vi "example-SetGetControlValue.vi"() -> ()   [LabVIEW 2020]
uses:
  SetGetControlValue.lvlib
panel:
  out "x = y? 2":bool
  out "x = y?":bool
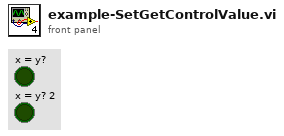
[diagram p1: front panel]
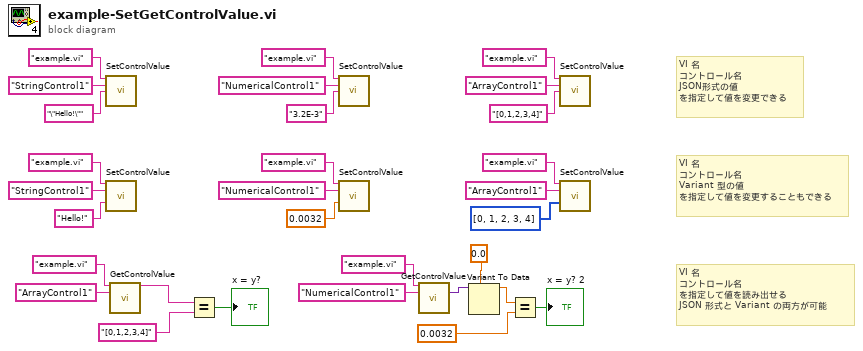
[diagram p0: block diagram]
diagram:
  # "VI 名\nコントロール名\nを指定して値を読み出せる\nJSON 形式と Variant の両方が可能"
  # "VI 名\nコントロール名\nVariant 型の値\nを指定して値を変更することもできる"
  # "VI 名\nコントロール名\nJSON形式の値\nを指定して値を変更できる"
  n1 = call "SetControlValue.vi"("vi"="example.vi", "ctrl"="StringControl1", "Value (JSON)"="\"Hello!\"") -> ()  [unwired: 12 in, 1 out]
  n2 = call "SetControlValue.vi"("vi"="example.vi", "ctrl"="StringControl1", "Value"="Hello!" ("Value (JSON)")) -> ()  [unwired: 12 in, 1 out]
  n3 = call "GetControlValue.vi"("vi"="example.vi", "ctrl"="ArrayControl1") -> ("String out"=w9:string)  [unwired: 11 in, 2 out]
  n4 = Equal?(x=w9, y="[0,1,2,3,4]" ("Value (JSON)")) -> (x = y?=→"x = y?":bool)
  n5 = call "SetControlValue.vi"("vi"="example.vi", "ctrl"="NumericalControl1", "Value (JSON)"="3.2E-3") -> ()  [unwired: 12 in, 1 out]
  n6 = call "SetControlValue.vi"("vi"="example.vi", "ctrl"="NumericalControl1", "Value"=0.0032 ("Value (JSON)")) -> ()  [unwired: 12 in, 1 out]
  n7 = call "GetControlValue.vi"("vi"="example.vi", "ctrl"="NumericalControl1") -> ("value"=w3:variant)  [unwired: 11 in, 2 out]
  n8 = Variant To Data(type=0.0 ("Value (JSON)"), Variant=w3) -> (data=w2:dbl)  [unwired: 1 in, 1 out]
  n9 = Equal?(x=w2, y=0.0032 ("Value (JSON)")) -> (x = y?=→"x = y? 2":bool)
  n10 = call "SetControlValue.vi"("vi"="example.vi", "ctrl"="ArrayControl1", "Value (JSON)"="[0,1,2,3,4]") -> ()  [unwired: 12 in, 1 out]
  n11 = call "SetControlValue.vi"("vi"="example.vi", "ctrl"="ArrayControl1", "Value"=i32[] [0, 1, 2, 3, 4] ("Value (JSON)")) -> ()  [unwired: 12 in, 1 out]
